vi "读取单点温度.vi"(8 "error in":errorcluster, 9 "y1":u16, 10 "x1":u16) -> (0 "error out":errorcluster, 2 "温度":dbl)   [LabVIEW 2016]
panel:
  out "data out":u8[](array[numeric])
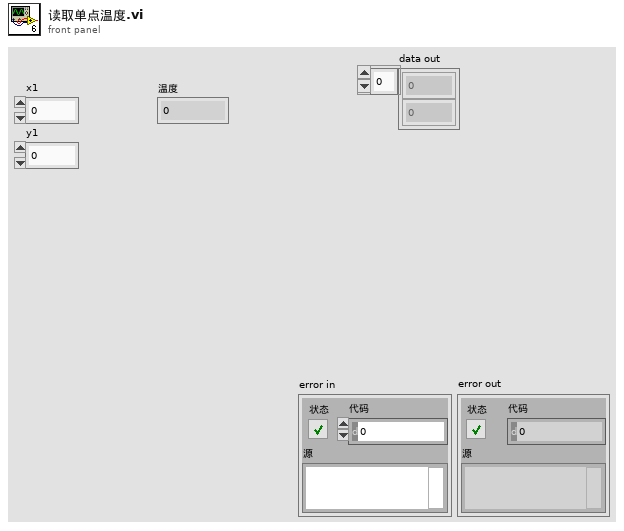
[diagram p1: front panel]
types:
  T1 = cluster{"byCmdType":u8, "bySubCmd":u8, "byParam_h":u8, "byParam_l":u8, "byAddr1_hh":u8, "byAddr1_h":u8, "byAddr1_l":u8, "byAddr1_ll":u8, "byAddr2_hh":u8, "byAddr2_h":u8, "byAddr2_l":u8, "byAddr2_ll":u8, "byLen_hh":u8, "byLen_h":u8, "byLen_l":u8, "byLen_ll":u8}
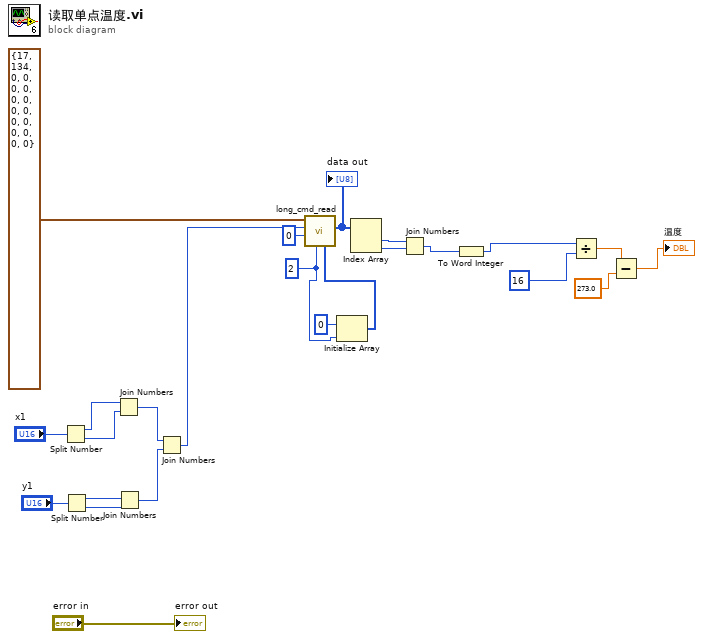
[diagram p0: block diagram]
diagram:
  w7 = u32 2 ("dwLen")
  n1 = Split Number(x="x1") -> (hi(x)=w21:u8, lo(x)=w20:u8)
  n2 = Split Number(x="y1") -> (hi(x)=w19:u8, lo(x)=w18:u8)
  n3 = Join Numbers(hi=w21, lo=w20) -> ((hi.lo)=w16:u16)
  n4 = Join Numbers(hi=w19, lo=w18) -> ((hi.lo)=w17:u16)
  n5 = Join Numbers(hi=w16, lo=w17) -> ((hi.lo)=w15:u32)
  n6 = Initialize Array(u8 0 ("element"), w7) -> (w6:u8[])
  n7 = call "long_cmd_read.vi"("data"=w6, "dwLen"=w7, "dwAddr2"=u32 0, "dwAddr1"=w15, "vd_cmd_long_header_t"=T1 {"byCmdType"=17, "bySubCmd"=134, "byParam_h"=0, "byParam_l"=0, "byAddr1_hh"=0, "byAddr1_h"=0, "byAddr1_l"=0, "byAddr1_ll"=0, "byAddr2_hh"=0, "byAddr2_h"=0, "byAddr2_l"=0, "byAddr2_ll"=0, "byLen_hh"=0, "byLen_h"=0, "byLen_l"=0, "byLen_ll"=0}) -> ("data out"=w13:u8[])  [unwired: 4 in, 2 out]
  "data out" <- w13
  n8 = Index Array(array=w13) -> (element #1=w12:u8, element #2=w11:u8)  [unwired: 2 in]
  n9 = Join Numbers(hi=w12, lo=w11) -> ((hi.lo)=w5:u16)
  n10 = To Word Integer(number=w5) -> (16bit integer=w4:i16)
  n11 = Divide(x=w4, y=u16 16) -> (x/y=w3:dbl)
  n12 = Subtract(x=w3, y=273.0) -> (x-y=→"温度":dbl)
  "error out" <- "error in"
